vi "WPI_CameraRead JPG.vi"(8 "error in":errorcluster, 9 "CGI?":bool=TRUE, 10 "fps":i32=10, 11 "address":string="192.168.1.101") -> (0 "error out":errorcluster, 3 "Raw Image Data":string)   [LabVIEW 2017]
doc: "This software is licensed. Open the labview\\readme\\WPI Robotics Library Open Source License.txt file for more information."
panel:
  out "Camera Request":string
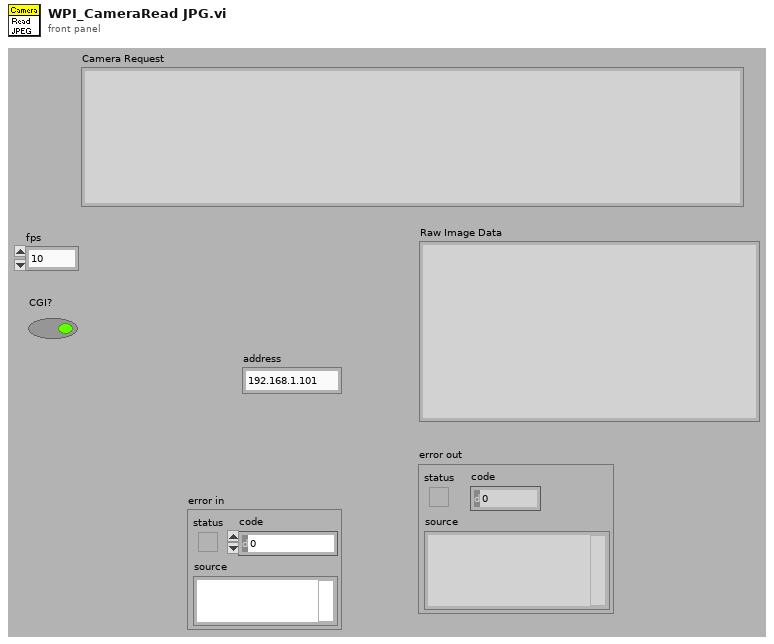
[diagram p1: front panel]
types:
  T1 = enum16{"Standard", "Buffered", "CRLF", "Immediate"}
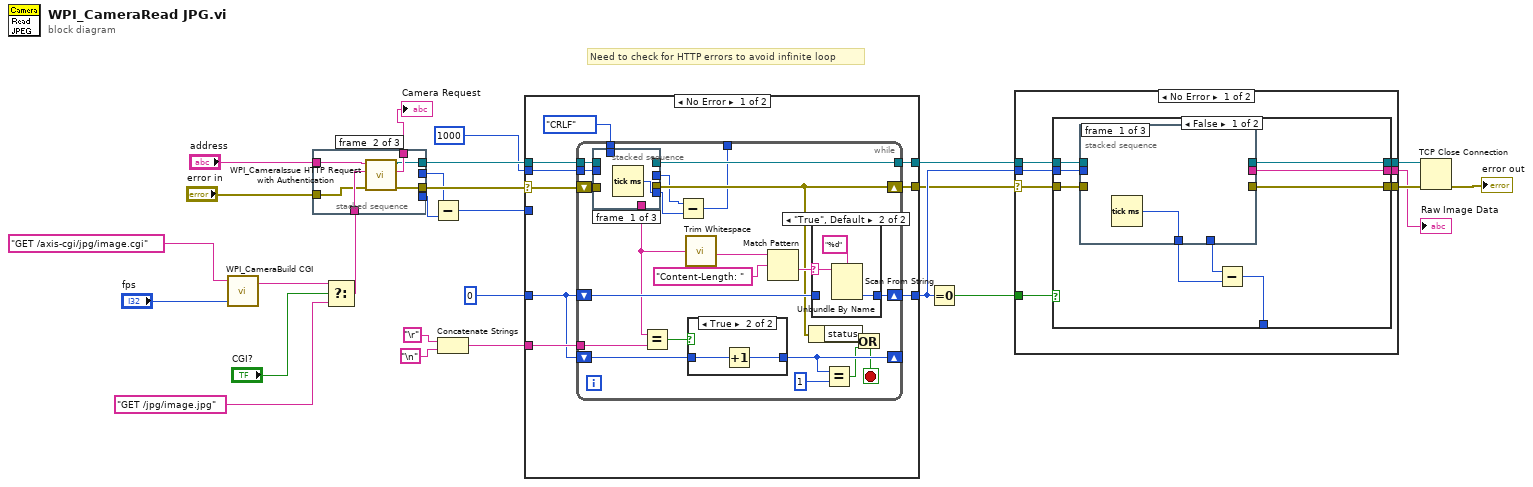
[diagram p0: block diagram]
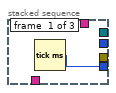
[diagram p2: hidden frame]
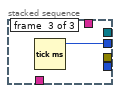
[diagram p3: hidden frame]
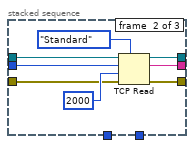
[diagram p4: hidden frame]
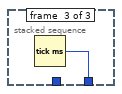
[diagram p5: hidden frame]
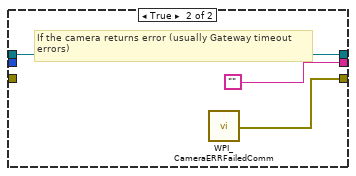
[diagram p6: hidden frame]
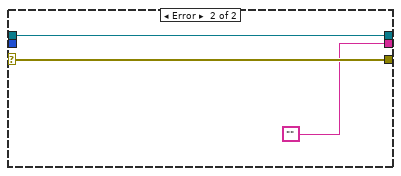
[diagram p7: hidden frame]
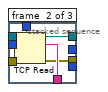
[diagram p8: hidden frame]
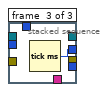
[diagram p9: hidden frame]
diagram:
  # "Need to check for HTTP errors to avoid infinite loop"
  n1 = call <vilib>:"WPI_CameraBuild CGI.vi"("fps"="fps", "Get String"="GET /axis-cgi/jpg/image.cgi") -> ("CGI String"=w23:string)  [unwired: 1 in, 1 out]
  n2 = Select(t=w23, s="CGI?", f="GET /jpg/image.jpg") -> (s? t:f=w17:string)
  n3 = stacked-sequence {
    tunnel: w17 -> [_ w34 _]
    tunnel: [_ w33 _] -> w15
    tunnel: [_ w32 _] -> w11
    tunnel: [_ w31 _] -> w10
    tunnel: "error in" -> [_ w30 _]
    tunnel: "address" -> [_ w29 _]
    tunnel: [w28 _ _] -> w2
    tunnel: [_ _ w35] -> w3
    frame #0 {
      n4 = Tick Count (ms)() -> (millisecond timer value=w28:u32)
    }
    frame #1 {
      n5 = call <vilib>:"WPI_CameraIssue HTTP Request with Authentication.vi"("error in (no error)"=w30, "Request"=w34, "address"=w29) -> ("error out"=w32:errorcluster, "Authenticated request"=w33:string, "connection ID (dup)"=w31:refnum<k5>)  [unwired: 2 in, 4 out]
    }
    frame #2 {
      n6 = Tick Count (ms)() -> (millisecond timer value=w35:u32)
    }
  }
  "Camera Request" <- w15
  n7 = Subtract(x=w3, y=w2) -> (x-y=w1:u32)
  n8 = Concatenate Strings("\r", "\n") -> (w20:string)
  n9 = case shown="No Error" w11 {
    selector: w11 -> [w36 w84]
    tunnel: [w44 w84] -> w8
    tunnel: [w43 w85] -> w13
    tunnel: [w42 w86] -> w12
    tunnel: w20 -> [w41 _]
    tunnel: 0 -> [w40 w85]
    tunnel: w10 -> [w38 w86]
    tunnel: 1000 ("bytes to read") -> [w37 _]
    tunnel: w1 -> [_ _]
    frame No Error {
      n10 = while {
        tunnel: w38 -> [w67]
        tunnel: [w66] -> w42
        shift-right: [w62] -> w43
        shift-left: w40 -> [w61]
        shift-right: [w58] -> _
        shift-left: w40 -> [w59]
        tunnel: w41 -> [w55]
        tunnel: w37 -> [w54]
        tunnel: T1."CRLF" ("mode (standard)") -> [w53]
        shift-right: [w51] -> w44
        shift-left: w36 -> [w52]
        tunnel: [w45] -> _
        stop <- w48 stop-if-true
        n11 = stacked-sequence {
          tunnel: w67 -> [_ w75 _]
          tunnel: [_ w74 _] -> w66
          tunnel: [_ w73 _] -> w56
          tunnel: w54 -> [_ w72 _]
          tunnel: w53 -> [_ w71 _]
          tunnel: w52 -> [_ w70 _]
          tunnel: [_ w69 _] -> w51
          tunnel: [w68 _ _] -> w46
          tunnel: [_ _ w76] -> w47
          frame #0 {
            n12 = Tick Count (ms)() -> (millisecond timer value=w68:u32)
          }
          frame #1 {
            n13 = TCP Read(connection ID=w75, bytes to read=w72, error in (no error)=w70, 7:w71) -> (connection ID out=w74:refnum<k5>, data out=w73:string, error out=w69:errorcluster)  [unwired: 1 out]
          }
          frame #2 {
            n14 = Tick Count (ms)() -> (millisecond timer value=w76:u32)
          }
        }
        n15 = Equal?(x=w56, y=w55) -> (x = y?=w60:bool)
        n16 = Subtract(x=w47, y=w46) -> (x-y=w45:u32)
        n17 = call <vilib>:"Trim Whitespace.vi"("string"=w56) -> ("trimmed string"=w64:string)  [unwired: 1 in]
        n18 = case shown="True" w60 {
          tunnel: w59 -> [w77 w79]
          tunnel: [w77 w78] -> w58
          frame False {
          }
          frame True {
            n19 = Increment(x=w79) -> (x+1=w78:i32)
          }
        }
        n20 = Match Pattern(string=w64, regular expression="Content-Length: ") -> (after substring=w63:string)  [unwired: 4 out]
        n21 = Unbundle By Name(w51) -> ("status"=w50:bool)
        n22 = case shown="\"True\", Default" w63 {
          selector: w63 -> [_ w82]
          tunnel: [w80 w83] -> w62
          tunnel: w61 -> [w80 _]
          frame "" {
          }
          frame "True", Default {
            n23 = Scan From String(format string="%d", input string=w82) -> (output 1=w83:i32)  [unwired: 2 in, 4 out]
          }
        }
        n24 = Equal?(x=w58, y=1) -> (x = y?=w49:bool)
        n25 = Or(x=w50, y=w49) -> (x .or. y?=w48:bool)
      }
    }
    frame Error {
    }
  }
  n26 = Equal To 0?(x=w13) -> (x = 0?=w14:bool)
  n27 = case shown="No Error" w8 {
    selector: w8 -> [w87 w118]
    tunnel: [w93 w118] -> w26
    tunnel: [w92 ""] -> w25
    tunnel: [w91 w116] -> w18
    tunnel: w14 -> [w90 _]
    tunnel: w13 -> [w89 _]
    tunnel: w12 -> [w88 w116]
    frame No Error {
      n28 = case shown="False" w90 {
        tunnel: w88 -> [w102 w114]
        tunnel: [w101 w113] -> w93
        tunnel: [w99 ""] -> w92
        tunnel: w89 -> [w100 _]
        tunnel: [w98 w114] -> w91
        tunnel: w87 -> [w97 _]
        tunnel: [w94 _] -> _
        frame False {
          n29 = stacked-sequence {
            tunnel: w102 -> [_ w111 _]
            tunnel: [_ w110 _] -> w101
            tunnel: w100 -> [_ w107 _]
            tunnel: [_ w106 _] -> w99
            tunnel: [_ w105 _] -> w98
            tunnel: w97 -> [_ w104 _]
            tunnel: [_ _ w112] -> w96
            tunnel: [w103 _ _] -> w95
            frame #0 {
              n30 = Tick Count (ms)() -> (millisecond timer value=w103:u32)
            }
            frame #1 {
              n31 = TCP Read(connection ID=w111, bytes to read=w107, error in (no error)=w104, 7:T1."Standard" ("mode (standard)"), 9:2000 ("timeout ms (25000)")) -> (connection ID out=w105:refnum<k5>, data out=w106:string, error out=w110:errorcluster)
            }
            frame #2 {
              n32 = Tick Count (ms)() -> (millisecond timer value=w112:u32)
            }
          }
          n33 = Subtract(x=w96, y=w95) -> (x-y=w94:u32)
        }
        frame True {
          # "If the camera returns error (usually Gateway timeout\nerrors)"
          n34 = call <vilib>:"WPI_CameraERRFailedComm.vi"() -> ("error out"=w113:errorcluster)
        }
      }
    }
    frame Error {
    }
  }
  "Raw Image Data" <- w25
  n35 = TCP Close Connection(connection ID=w18, error in (no error)=w26) -> (error out=→"error out":errorcluster)  [unwired: 2 out]
